vi "DAQmx Read (Digital 1D U8 NChan 1Samp).vi"(0 "task/channels in":refnum<k21>, 9 "timeout":dbl=10.0 format="%0.2f", 11 "error in":errorcluster) -> (4 "task out":refnum<k21>, 6 "data":u8[](array[numeric]), 15 "error out":errorcluster)   [LabVIEW 2011]
doc: "Reads a single 8-bit unsigned integer sample from each channel in a task that contains one or more digital input channels. Use an instance that reads 8-bit unsigned integers for devices with up to eight lines per port."
uses:
  nilvaiu.dll
panel:
  # "channel"
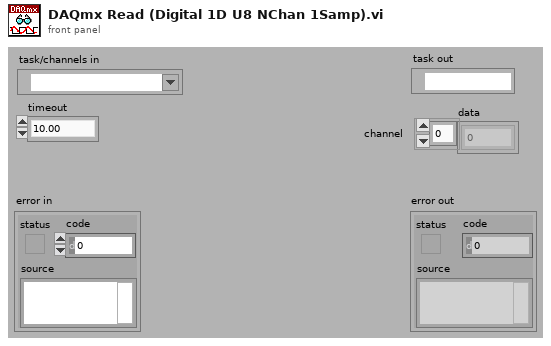
[diagram p1: front panel]
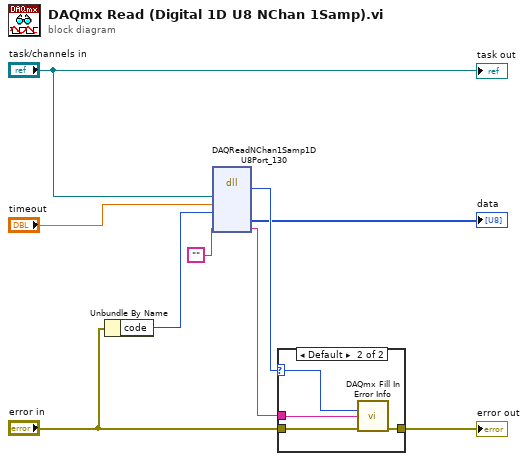
[diagram p0: block diagram]
diagram:
  n1 = Unbundle By Name("error in") -> ("code"=w3:i32)
  n2 = dll-call lib="nilvaiu.dll" fn="DAQReadNChan1Samp1DU8Port_130"("taskID"="task/channels in", "timeout"="timeout", "incomingStatus"=w3, "extendedErrorInfo"="") -> (w7:i32, "data"=→"data":u8[], "extendedErrorInfo"=w2:string)  [unwired: 6 in, 3 out]
  n3 = case shown="Default" w7 {
    selector: w7 -> [_ w12]
    tunnel: "error in" -> [w10 w14]
    tunnel: [w10 w13] -> w9
    tunnel: w2 -> [_ w11]
    frame 0 {
    }
    frame Default {
      n4 = call "DAQmx Fill In Error Info.vi"("status code"=w12, "extended error info"=w11, "error in"=w14) -> ("error out"=w13:errorcluster)  [unwired: 1 in, 11 out]
    }
  }
  "error out" <- w9
  "task out" <- "task/channels in"
